vi "GetPositionDetails.vi"(8 "error in (no error)":errorcluster, 9 "Seperator in":string, 10 "Command":string, 11 "Picomotor8752 in":refnum<class "Picomotor8742.lvclass">) -> (0 "error out":errorcluster, 1 "DeviceOut":string, 2 "AxisNumber":u32, 3 "Picomotor8752 Out":refnum<class "Picomotor8742.lvclass">, 4 "RelativeMovement":i32, 6 "AbsolutePosition":i32)   [LabVIEW 2020, in "Picomotor8742.lvclass"]
uses:
  Picomotor8742.lvclass
  Picomotor8742.lvclass/Picomotor8742.ctl
  shared/UtilsLib/ClusterManipulation/GetClusterElementByName(I32).vi
  ESP301/ESP301.lvclass
  shared/UtilsLib/ClusterManipulation/GetClusterElementByName.lvlib
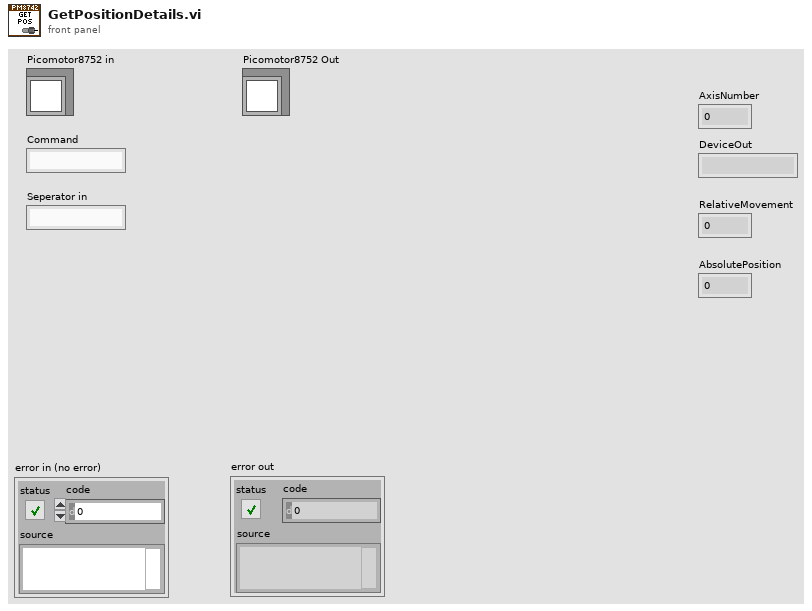
[diagram p1: front panel]
types:
  T1 = cluster{"device 1":cluster{"Value":dbl, "Min":dbl, "Max":dbl, "StepSize":dbl, "Tolerance":dbl, "ValueActual":dbl}, "device 2":cluster{"Value":dbl, "Min":dbl, "Max":dbl, "StepSize":dbl, "Tolerance":dbl, "ValueActual":dbl}, "device 3":cluster{"Value":dbl, "Min":dbl, "Max":dbl, "StepSize":dbl, "Tolerance":dbl, "ValueActual":dbl}, "device 4":cluster{"Value":dbl, "Min":dbl, "Max":dbl, "StepSize":dbl, "Tolerance":dbl, "ValueActual":dbl}}
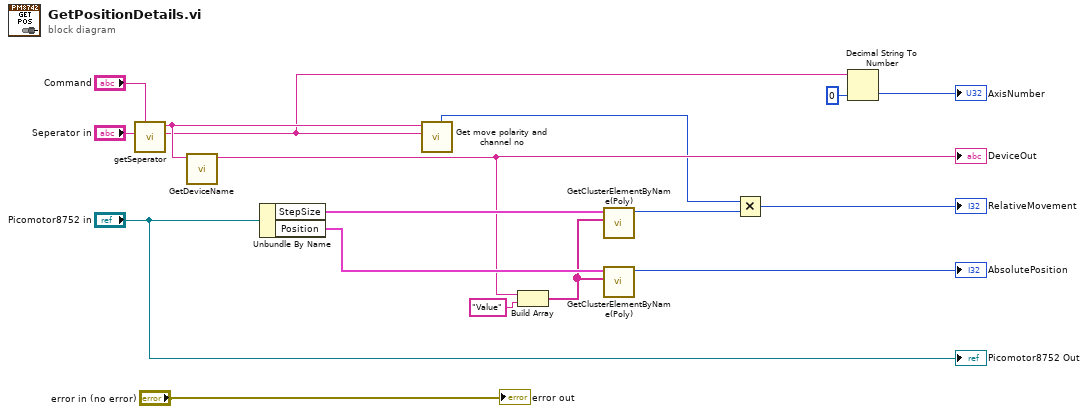
[diagram p0: block diagram]
diagram:
  n1 = call "getSeperator.vi"("Channel Seperator (\"\")"="Seperator in", "Command"="Command") -> ("Channel"=w3:string, "Seperator (e.g. \"Channel1\")"=w9:string)  [unwired: 8 in]
  n2 = call "GetDeviceName.vi"("Seperator (e.g. \"Channel1\")"=w9) -> ("String"=w14:string)  [unwired: 10 in]
  "DeviceOut" <- w14
  n3 = Unbundle By Name("Picomotor8752 in") -> ("StepSize"=w17:T1, "Position"=w16:T1)
  n4 = call "Get move polarity and channel no.vi"("Channel in"=w3, "Channel string In"=w9) -> ("Numeric"=w10:i32)  [unwired: 7 in, 2 out]
  n5 = Build Array(w14, "Value" ("string")) -> (w15:string[])
  n6 = call-poly "GetClusterElementByName(Poly).vi"("ElementName"=w15, "Cluster"=w17) -> ("ValueOut"=w12:i32)  [unwired: 8 in, 1 out]
  n7 = call-poly "GetClusterElementByName(Poly).vi"("ElementName"=w15, "Cluster"=w16) -> ("ValueOut"=→"AbsolutePosition":i32)  [unwired: 8 in, 1 out]
  n8 = Multiply(x=w10, y=w12) -> (x*y=→"RelativeMovement":i32)
  n9 = Decimal String To Number(string=w3, default (0L)=u32 0 ("default (0 I32)")) -> (number=→"AxisNumber":u32)  [unwired: 1 in, 1 out]
  "Picomotor8752 Out" <- "Picomotor8752 in"
  "error out" <- "error in (no error)"
